vi "Hardware in the Loop - Upload Waveforms (Multiplexed - Signed 16 Bit).vi"(8 "error in":errorcluster, 10 "Multichannel Waveform":i16[][](array[numeric]), 11 "Configuration Cluster":T1={"Name"="Default Settings", "IP"="192.168.0.84", "Control Port"=4220, "Timeout (ms)"=2000, "Continuous Capture Port (Multiplexed)"=4210, "Start HIL Shot Port"=53999, "AWG Upload Port (Multiplexed)"=54201, "Download Captured Data Port (Multiplexed)"=53000, "Module Slots"=2, "Module Configurations"=[{"Name"="ACQ 425 ELF", "Position"="192.168.0.84", "Module Type"=enum."Analog In Module", "Control Port"=4221, "Timeout (ms)"=2000, "Channels"=16}, {"Name"="AO 424 ELF", "Position"="192.168.0.84", "Module Type"=enum."Analog Out Module", "Control Port"=4222, "Timeout (ms)"=2000, "Channels"=16}]}) -> (0 "error out":errorcluster)   [LabVIEW 2017, in "Communications Library.lvlib"]
doc: "Uploads a multichannel waveform to the DTACQ device.\n\nInitialises the connection, converts the data to a byte array, uploads the data and then closes the TCP connection."
uses:
  Communications Library.lvlib
  Typedefs/DTACQ Module Carrier Configuration--Cluster.ctl
  Typedefs/DTACQ Module Configuration--Cluster.ctl
  Typedefs/DTACQ Device Type--Enum.ctl
  Typedefs/Functional Global Variable Action--Enum.ctl
panel:
  out "millisecond timer":u32
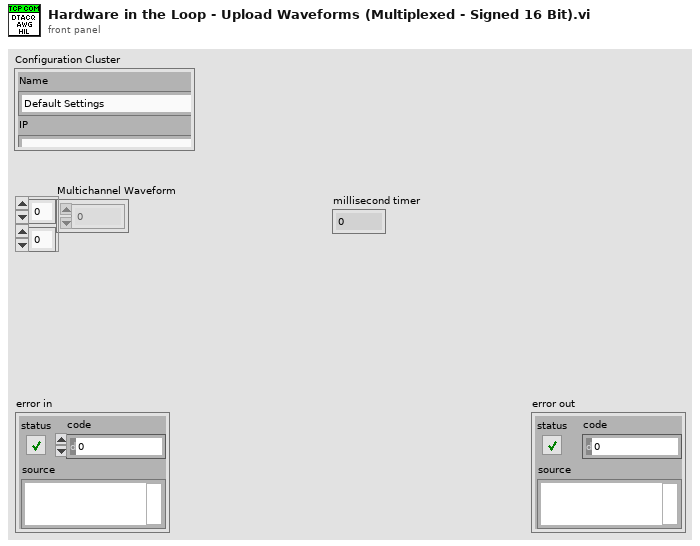
[diagram p1: front panel]
types:
  T1 = typedef "Communications Library.lvlib/DTACQ Module Carrier Configuration--Cluster.ctl" = cluster{"Name":string, "IP":string, "Control Port":i32, "Timeout (ms)":i32, "Continuous Capture Port (Multiplexed)":i32, "Start HIL Shot Port":i32, "AWG Upload Port (Multiplexed)":i32, "Download Captured Data Port (Multiplexed)":i32, "Module Slots":i32, "Module Configurations":T2[]}
  T2 = typedef "Communications Library.lvlib/DTACQ Module Configuration--Cluster.ctl" = cluster{"Name":string, "Position":string, "Module Type":T3, "Control Port":i32, "Timeout (ms)":i32, "Channels":i32}
  T3 = typedef "Communications Library.lvlib/DTACQ Device Type--Enum.ctl" = enum16{"Carrier", "Analog In Module", "Analog Out Module", "Generic Module"}
  T4 = typedef "Communications Library.lvlib/Functional Global Variable Action--Enum.ctl" = enum16{"Initialise", "Write Module Config", "Write Carrier Config", "Read"}
  T5 = typedef "Communications Library.lvlib/DTACQ Connection Data--Cluster.ctl" = cluster{"Description":string, "Address":string, "Port":u16, "timeout (ms)":i32, "Termination Character":string, "TCP Connection Reference":refnum<k5>, "Open Connection":bool}
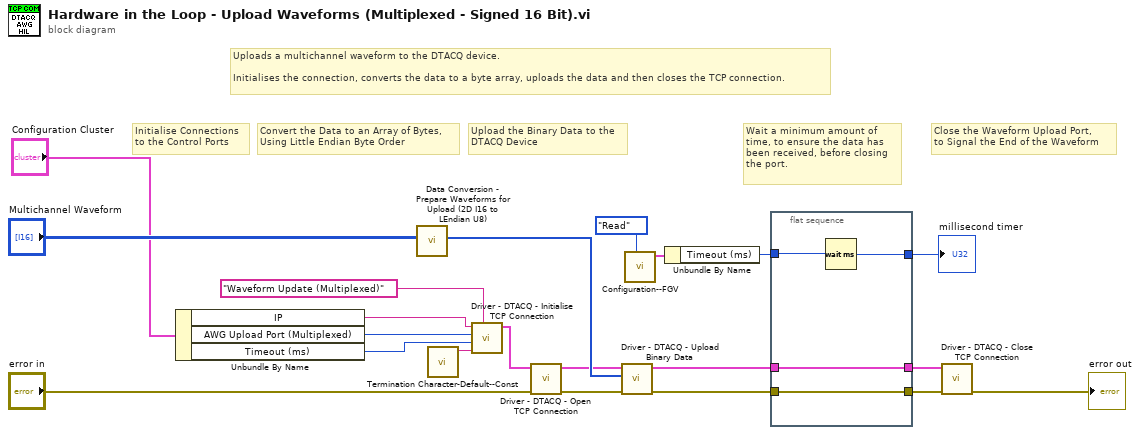
[diagram p0: block diagram]
diagram:
  # "Uploads a multichannel waveform to the DTACQ device.\n\nInitialises the connection, converts the data to a byte array, uploads the data and then closes the TCP connection."
  # "Wait a minimum amount of\ntime, to ensure the data has\nbeen received, before closing\nthe port."
  # "Close the Waveform Upload Port,\nto Signal the End of the Waveform"
  # "Upload the Binary Data to the\nDTACQ Device"
  # "Convert the Data to an Array of Bytes,\nUsing Little Endian Byte Order"
  # "Initialise Connections\nto the Control Ports"
  n1 = Unbundle By Name("Configuration Cluster") -> ("IP"=w1:string, "AWG Upload Port (Multiplexed)"=w7:i32, "Timeout (ms)"=w6:i32)
  n2 = call "Data Conversion - Prepare Waveforms for Upload (2D I16 to LEndian U8).vi"("Multichannel Waveform (Signed 16 Bit - 2D Array)"="Multichannel Waveform") -> ("Unsigned Byte Array"=w20:u8[])  [unwired: 10 in]
  n3 = call "Termination Character-Default--Const.vi"() -> ("Termination Character"=w16:string)  [unwired: 11 in]
  n4 = call "Driver - DTACQ - Initialise TCP Connection.vi"("Description"="Waveform Update (Multiplexed)", "Termination Character"=w16, "timeout (ms)"=w6, "Port"=w7, "Address"=w1) -> ("DTACQ Connection Data Out"=w19:T5)  [unwired: 6 in]
  n5 = call "Driver - DTACQ - Open TCP Connection.vi"("error in"="error in", "DTACQ Connection Data In"=w19) -> ("error out"=w14:errorcluster, "DTACQ Connection Data Out"=w15:T5)  [unwired: 8 in]
  n6 = call "Driver - DTACQ - Upload Binary Data.vi"("error in"=w14, "Unsigned Byte Array"=w20, "DTACQ Connection Data In"=w15) -> ("error out"=w11:errorcluster, "DTACQ Connection Data Out"=w12:T5)  [unwired: 7 in]
  n7 = call "Configuration--FGV.vi"("Functional Global Action"=Functional_Global_Variable_Action--Enum."Read") -> ("Carrier Configuration Out"=w4:T1)  [unwired: 9 in, 1 out]
  n8 = Unbundle By Name(w4) -> ("Timeout (ms)"=w3:i32)
  n9 = flat-sequence {
    tunnel: w3 -> [w23]
    tunnel: w12 -> [w24]
    tunnel: w11 -> [w25]
    tunnel: [w25] -> w10
    tunnel: [w24] -> w9
    tunnel: [w22] -> w8
    frame #0 {
      n10 = Wait (ms)(milliseconds to wait=w23) -> (millisecond timer value=w22:u32)
    }
  }
  n11 = call "Driver - DTACQ - Close TCP Connection.vi"("error in"=w10, "DTACQ Connection Data In"=w9) -> ("error out"=→"error out":errorcluster)  [unwired: 8 in, 1 out]
  "millisecond timer" <- w8
